vi "Centauro LED Low Level Parser Dryer.vi"(8 "error in (no error)":errorcluster, 9 "Read ERD List":T3[](array[typedef])=[{"ERD Number"=61758, "Data Type"=enum."string"}, {"ERD Number"=61755, "Data Type"=enum."string"}, {"ERD Number"=61757, "Data Type"=enum."string"}, {"ERD Number"=61756, "Data Type"=enum."string"}, {"ERD Number"=61751, "Data Type"=enum."string"}] {"ERD Number" format="%.0x"}, 10 "Raw Data In":string) -> (0 "error out":errorcluster, 1 "Binary Number":u32, 2 "LED Status":T2)   [LabVIEW 2016]
uses:
  Common/LabVIEW GEA2 Toolkit/LabVIEW_GEA2_Toolkit.lvlibp/type defs/ERD Read Data In.ctl
  Common/LabVIEW GEA2 Toolkit/LabVIEW_GEA2_Toolkit.lvlibp/type defs/Data Type.ctl
  Centauro Washer/Product Testcode/Centauro/Valew Common/type defs/LED Status OOB.ctl
  Common/LabVIEW GEA2 Toolkit/LabVIEW_GEA2_Toolkit.lvlibp
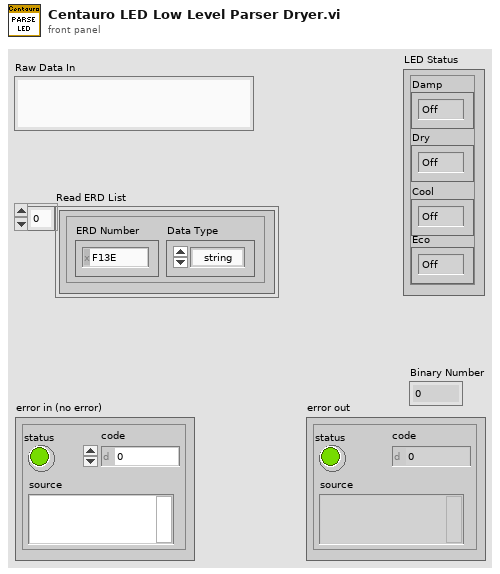
[diagram p1: front panel]
types:
  T1 = typedef "LED Status OOB.ctl" = enum32{"Off", "On", "Blink"}
  T2 = cluster{"Damp":T1, "Dry":T1, "Cool":T1, "Eco":T1}
  T3 = typedef "LabVIEW_GEA2_Toolkit.lvlibp/ERD Read Data In.ctl" = cluster{"ERD Number":u16, "Data Type":T4}
  T4 = typedef "LabVIEW_GEA2_Toolkit.lvlibp/Data Type.ctl" = enum16{"string", "boolean", "uint8_t", "uint16_t", "uint32_t", "uint64_t", "int8_t", "int16_t", "int32_t", "int64_t"}
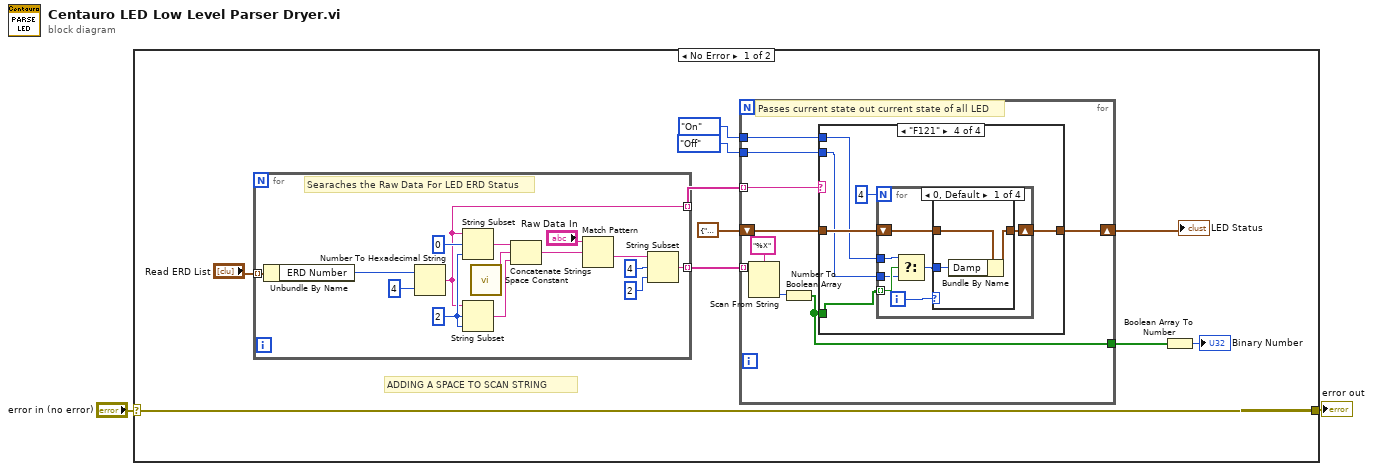
[diagram p0: block diagram]
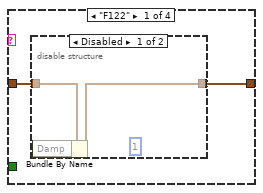
[diagram p2: hidden frame]
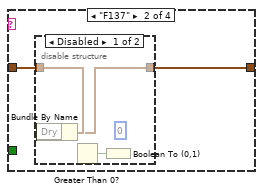
[diagram p4: hidden frame]
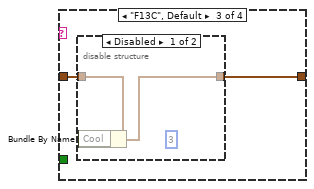
[diagram p6: hidden frame]
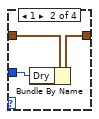
[diagram p8: hidden frame]
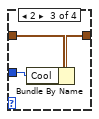
[diagram p9: hidden frame]
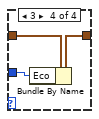
[diagram p10: hidden frame]
diagram:
  n1 = case shown="No Error" "error in (no error)" {
    selector: "error in (no error)" -> [w9 w75]
    tunnel: [w9 w75] -> w1
    frame No Error {
      # "ADDING A SPACE TO SCAN STRING"
      n2 = for {
        tunnel: "Read ERD List" -> [w27] mode=indexing
        tunnel: [w21] -> w11 mode=indexing
        tunnel: [w17] -> w10 mode=indexing
        w19 = 2 ("offset (0)")
        # "Searaches the Raw Data For LED ERD Status"
        n3 = Unbundle By Name(w27) -> ("ERD Number"=w25:u16)
        n4 = Number To Hexadecimal String(1:i16 4 ("width (-)"), 2:w25) -> (0:w17:string)
        n5 = String Subset(string=w17, offset (0)=0 ("length (rest)"), length (rest)=w19) -> (substring=w16:string)
        n6 = String Subset(string=w17, offset (0)=w19, length (rest)=w19) -> (substring=w20:string)
        n7 = call <vilib>:"Space Constant.vi"() -> ("String"=w15:string)
        n8 = Concatenate Strings(w16, w15, w20) -> (w14:string)
        n9 = Match Pattern(string="Raw Data In", regular expression=w14) -> (after substring=w22:string)  [unwired: 1 in, 3 out]
        n10 = String Subset(string=w22, offset (0)=4 ("length (rest)"), length (rest)=2 ("offset (0)")) -> (substring=w21:string)
      }
      n11 = for {
        shift-right: [w35] -> w7
        shift-left: T2 {"Damp"=enum."Off", "Dry"=enum."Off", "Cool"=enum."Off", "Eco"=enum."Off"} ("LED Status") -> [w36]
        tunnel: w11 -> [w33] mode=indexing
        tunnel: w10 -> [w32] mode=indexing
        tunnel: LED_Status_OOB."Off" ("Damp") -> [w31]
        tunnel: LED_Status_OOB."On" ("Damp") -> [w30]
        tunnel: [w28] -> w3
        # "Passes current state out current state of all LED"
        n12 = Scan From String(format string="%X", input string=w33) -> (output 1=w29:u32)  [unwired: 3 in, 3 out]
        n13 = Number To Boolean Array(number=w29) -> (Boolean array=w28:bool[])
        n14 = case shown="\"F121\"" w32 {
          tunnel: w36 -> [w38 w42 w47 w55]
          tunnel: [w37 w41 w46 w54] -> w35
          tunnel: w31 -> [_ _ _ w53]
          tunnel: w30 -> [_ _ _ w52]
          tunnel: w28 -> [_ _ _ w51]
          frame "F122" {
            n15 = disable-structure shown="Disabled" {
              disable-tunnel: w38 -> [w40 _]
              disable-tunnel: [w39 _] -> w37
              frame Disabled {
                (unwired) 1 ("index")
                n16 = Bundle By Name(cluster=w40) -> (w39:T2)  [unwired: 1 in]
              }
              frame Enabled {
              }
            }
          }
          frame "F137" {
            n17 = disable-structure shown="Disabled" {
              disable-tunnel: w42 -> [w45 _]
              disable-tunnel: [w44 _] -> w41
              frame Disabled {
                (unwired) 0 ("index")
                n18 = Bundle By Name(cluster=w45) -> (w44:T2)  [unwired: 1 in]
                n19 = Greater Than 0?() -> (x > 0?=w43:bool)  [unwired: 1 in]
                n20 = Boolean To (0,1)(Boolean=w43) -> ()  [unwired: 1 out]
              }
              frame Enabled {
              }
            }
          }
          frame "F13C", Default {
            n21 = disable-structure shown="Disabled" {
              disable-tunnel: w47 -> [w49 _]
              disable-tunnel: [w48 _] -> w46
              frame Disabled {
                (unwired) 3 ("index")
                n22 = Bundle By Name(cluster=w49) -> (w48:T2)  [unwired: 1 in]
              }
              frame Enabled {
              }
            }
          }
          frame "F121" {
            n23 = for {
              N: 4 -> [_]
              shift-right: [w61] -> w54
              shift-left: w55 -> [w62]
              tunnel: w51 -> [w59] mode=indexing
              tunnel: w53 -> [w58]
              tunnel: w52 -> [w57]
              i -> [w60]
              n24 = Select(t=w57, s=w59, f=w58) -> (s? t:f=w56:T1)
              n25 = case shown="0, Default" w60 {
                tunnel: w62 -> [w64 w68 w71 w74]
                tunnel: [w63 w67 w70 w73] -> w61
                tunnel: w56 -> [w65 w66 w69 w72]
                frame 0, Default {
                  n26 = Bundle By Name(cluster=w64, "Damp"=w65) -> (w63:T2)
                }
                frame 1 {
                  n27 = Bundle By Name(cluster=w68, "Dry"=w66) -> (w67:T2)
                }
                frame 2 {
                  n28 = Bundle By Name(cluster=w71, "Cool"=w69) -> (w70:T2)
                }
                frame 3 {
                  n29 = Bundle By Name(cluster=w74, "Eco"=w72) -> (w73:T2)
                }
              }
            }
          }
        }
      }
      "LED Status" <- w7
      n30 = Boolean Array To Number(Boolean array=w3) -> (number=→"Binary Number":u32)
    }
    frame Error {
    }
  }
  "error out" <- w1
